vi "Keyence.Main-Destructor.vi"(7 "Idx":i32, 8 "error in":errorcluster) -> (0 "error out":errorcluster)   [LabVIEW 2015]
uses:
  Keyence.Action.ctl
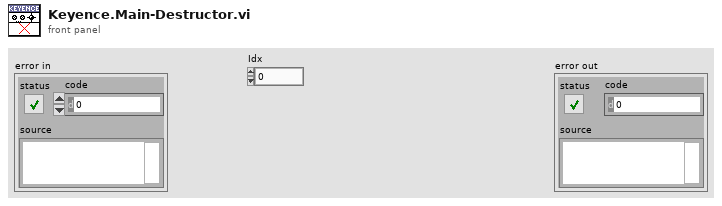
[diagram p1: front panel]
types:
  T1 = typedef "Keyence.Action.ctl" = enum32{"idle", "constructor", "destructor", "--- Keyence ---", "Init", "Scan"}
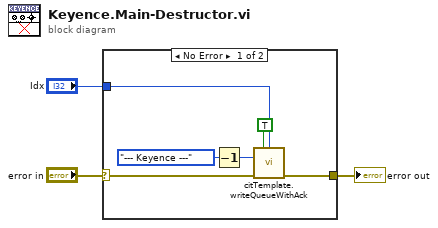
[diagram p0: block diagram]
diagram:
  n1 = case shown="No Error" "error in" {
    selector: "error in" -> [w9 w10]
    tunnel: [w8 w10] -> w2
    tunnel: "Idx" -> [w4 _]
    frame No Error {
      n2 = Decrement(x=Keyence.Action."--- Keyence ---" ("Action")) -> (x-1=w5:T1)
      n3 = call "citTemplate.writeQueueWithAck.vi"("High priority (F)"=TRUE, "instance (0)"=w4, "event in"=w5, "error in (no error)"=w9) -> ("error out"=w8:errorcluster)  [unwired: 9 in, 2 out]
    }
    frame Error {
    }
  }
  "error out" <- w2
